vi "Set Tx Format.vi"(6 "Delimitated Char":string=".", 8 "error in (no error)":errorcluster, 9 "node status":T3 items=["Good"=0, "Uncertain"=1073741824, "Uncertain_InitialValue"=1083310080, "Uncertain_LastUsableValue"=1083179008, "Uncertain_SensorNotAccurate"=1083375616, "Uncertain_EngineeringUnitsExceeded"=1083441152, "Bad"=2147483648, "Bad_NoCommunication"=2150694912, "Bad_NotReadable"=2151284736, "Bad_NotWritable"=2151350272, "Bad_OutOfRange"=2151415808, "Bad_WaitingForInitialData"=2150760448], 10 "NodeIDs":string[](array[string]), 11 "Controls":refnum<vi>[](array[refnum])) -> (0 "error out":errorcluster, 3 "Dataset":T1[](array[typedef]) {"node status" items=["Good"=0, "Uncertain"=1073741824, "Uncertain_InitialValue"=1083310080, "Uncertain_LastUsableValue"=1083179008, "Uncertain_SensorNotAccurate"=1083375616, "Uncertain_EngineeringUnitsExceeded"=1083441152, "Bad"=2147483648, "Bad_NoCommunication"=2150694912, "Bad_NotReadable"=2151284736, "Bad_NotWritable"=2151350272, "Bad_OutOfRange"=2151415808, "Bad_WaitingForInitialData"=2150760448]})   [LabVIEW 2021, in "OPCUA.lvlib"]
uses:
  <vilib>/OPCUA/controls/Write Status.ctl
  <vilib>/OPCUA/controls/Write Variant Request.ctl
  <vilib>/OPCUA/controls/NodeId.ctl
  OPCUA.lvlib
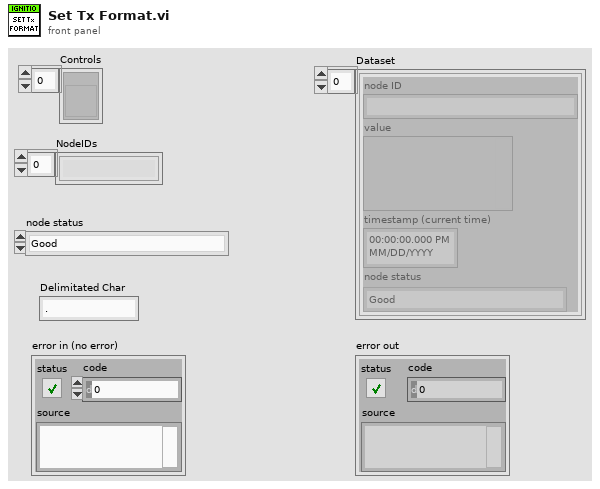
[diagram p1: front panel]
types:
  T1 = typedef "Write Variant Request.ctl" = cluster{"node ID":T2, "value":variant, "timestamp (current time)":timestamp, "node status":T3}
  T2 = typedef "NodeId.ctl" = string
  T3 = typedef "Write Status.ctl" = u32
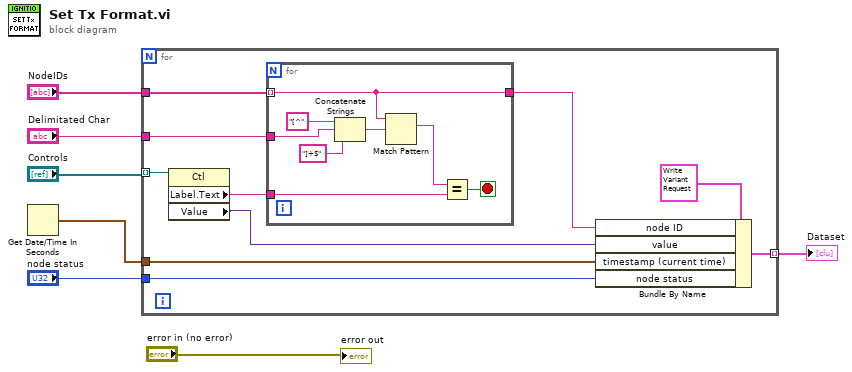
[diagram p0: block diagram]
diagram:
  n1 = Get Date/Time In Seconds() -> (seconds since 1Jan1904=w7:timestamp)
  n2 = for {
    tunnel: "Controls" -> [w17] mode=indexing
    tunnel: [w13] -> w3 mode=indexing
    tunnel: w7 -> [w12]
    tunnel: "NodeIDs" -> [w15]
    tunnel: "node status" -> [w10]
    tunnel: "Delimitated Char" -> [w8]
    n3 = property class="Ctl"(reference=w17) -> ("Label.Text"=w16:string, "Value"=w9:variant)  [unwired: 1 in, 2 out]
    n4 = for {
      tunnel: w16 -> [w25]
      tunnel: w15 -> [w20] mode=indexing
      tunnel: [w20] -> w11
      tunnel: w8 -> [w19]
      stop <- w24 stop-if-true
      n5 = Concatenate Strings("[^" ("string"), w19, "]+$" ("string")) -> (w23:string)
      n6 = Match Pattern(string=w20, regular expression=w23) -> (match substring=w18:string)  [unwired: 1 in, 3 out]
      n7 = Equal?(x=w18, y=w25) -> (x = y?=w24:bool)
    }
    n8 = Bundle By Name(cluster=T1 {"node ID"="", "value"=variant, "timestamp (current time)"=timestamp(0 s since 1904-01-01), "node status"=0} ("request"), "node ID"=w11, "value"=w9, "timestamp (current time)"=w12, "node status"=w10) -> (w13:T1)
  }
  "Dataset" <- w3
  "error out" <- "error in (no error)"
